vi "Configure Standard Waveform Amp Only.vi"(0 "VISA resource name":refnum<visa-resource-name>, 2 "Channel (1:Channel 1)":i32(ring)=1 items=["Channel 1"=1, "Channel 2"=2], 5 "Amplitude (1.0 Vpp)":dbl=1.0 min=0.001 max=20.0 step=1.0 format="%#.3f", 7 "Delay Time (600)":u32=600, 11 "error in (no error)":errorcluster) -> (4 "VISA resource name out":refnum<visa-resource-name>, 15 "error out":errorcluster)   [LabVIEW 2017, in "Siglent SDG 1000 5000 800 Series.lvlib"]
doc: "Selects the waveform shape, frequency, amplitude, offset, and phase for standard waveforms (including Sine, Square, Ramp, Pulse, DC and Arb).\n\nNotes: To configure other parameters for pulse waveforms please run the Configure Pulse VI. \nTo configure noise waveforms please run the Configure Noise VI.\nTo configure other parameters for arbitrary waveforms please run the Create Arbitrary Waveform."
uses:
  <instrlib>/Siglent SDG 1000 5000 800 Series/Siglent SDG 1000 5000 800 Series.lvlib
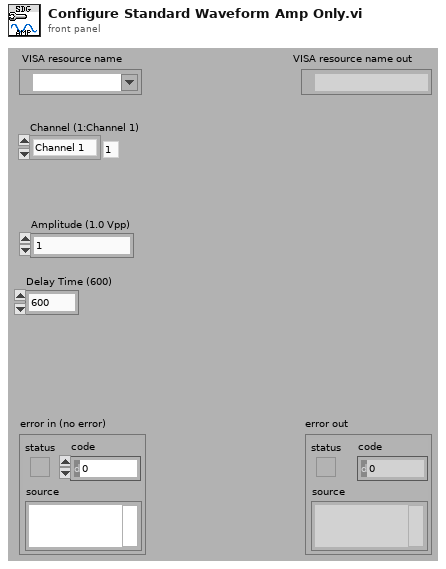
[diagram p1: front panel]
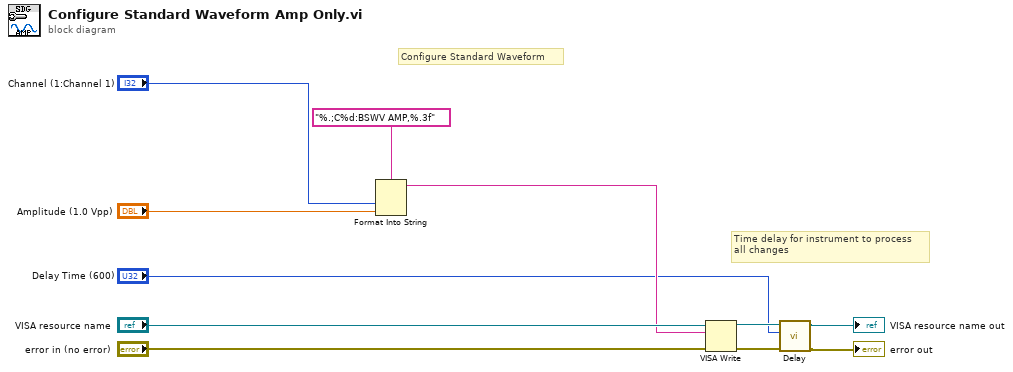
[diagram p0: block diagram]
diagram:
  # "Time delay for instrument to process\nall changes"
  # "Configure Standard Waveform"
  n1 = Format Into String(format string="%.;C%d:BSWV AMP,%.3f", "Channel (1:Channel 1)", "Amplitude (1.0 Vpp)") -> (resulting string=w3:string)  [unwired: 2 in, 1 out]
  n2 = VISA Write(VISA resource name="VISA resource name", write buffer=w3, error in (no error)="error in (no error)") -> (VISA resource name out=w8:refnum<visa-resource-name>, error out=w7:errorcluster)  [unwired: 1 out]
  n3 = call <instrlib>:"Delay.vi"("error in (no error)"=w7, "Delay Time (600)"="Delay Time (600)", "VISA resource name"=w8) -> ("error out"=→"error out":errorcluster, "VISA resource name out"=→"VISA resource name out":refnum<visa-resource-name>)  [unwired: 7 in]
